vi "SMSD_CODE_CMD_REQUEST_cmd.vi"(8 "error in (no error)":errorcluster, 10 "Password":string="0123456789ABCDEF", 11 "SMSD in":refnum<class "SMSD Master.lvclass">) -> (0 "error out":errorcluster, 1 "PDU valid?":bool, 3 "SMSD out":refnum<class "SMSD Master.lvclass">)   [LabVIEW 2021, in "SMSD Master.lvclass"]
uses:
  SMSD Master.lvclass
  Data Unit/SMSD Data Unit/ERROR_OR_COMMANT_Type.ctl
  Data Unit/SMSD Data Unit/SMSD Data Unit.lvclass/SMSD Data Unit.ctl
  SMSD Master.lvclass/SMSD Master.ctl
  Transmission Data Unit/SMSD/SMSD ADU.lvclass/SMSD ADU.ctl
  Transmission Data Unit/SMSD/Write ADU Packet.vi
  Transmission Data Unit/SMSD/Read ADU Packet.vi
  Modbus_v121c/Network Interface/TCP Interface/TCP Shared Components/TCP Write.vi
  Data Unit/SMSD Data Unit/Flatten PDU.vi
  Data Unit/SMSD Data Unit/Unflatten to PDU.vi
  Modbus_v121c/Network Interface/TCP Interface/TCP Shared Components/TCP Read.vi
  <vilib>/Utility/error.llb/Clear Errors.vi
  Data Unit/SMSD Data Unit/SMSD Data Unit.lvclass
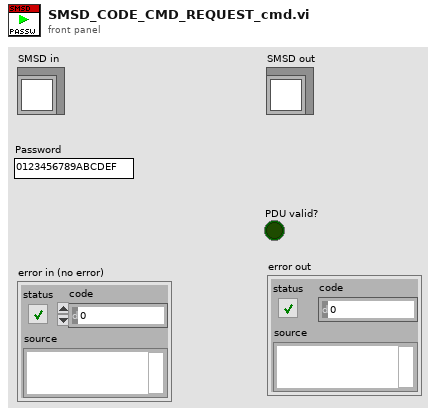
[diagram p1: front panel]
types:
  T1 = typedef "SMSD Data Unit.lvclass/ERROR_OR_COMMANT_Type.ctl" = enum8{"OK", "OK_ACCESS", "ERROR_ACCESS", "ERROR_ACCESS_TIMEOUT", "ERROR_XOR", "ERROR_NO_COMMAND", "ERROR_LEN", "ERROR_RANGE", "ERROR_WRITE", "ERROR_READ", "ERROR_PROGRAMS", "ERROR_WRITE_SETUP", "NO_NEXT", "END_PROGRAMS", "COMMAND_GET_STATUS_IN_EVENT", "COMMAND_GET_MODE", "COMMAND_GET_ABS_POS", "COMMAND_GET_EL_POS", "COMMAND_GET_SPEED", "COMMAND_GET_MIN_SPEED", "COMMAND_GET_MAX_SPEED", "COMMAND_GET_STACK", "STATUS_RELE_SET", "STATUS_RELE_CLR"}
  T2 = enum8{"CODE_CMD_REQUEST", "CODE_CMD_RESPONSE", "CODE_CMD_POWERSTEP01", "CODE_CMD_POWERSTEP01_W_MEM0", "CODE_CMD_POWERSTEP01_W_MEM1", "CODE_CMD_POWERSTEP01_W_MEM2", "CODE_CMD_POWERSTEP01_W_MEM3", "CODE_CMD_POWERSTEP01_R_MEM0", "CODE_CMD_POWERSTEP01_R_MEM1", "CODE_CMD_POWERSTEP01_R_MEM2", "CODE_CMD_POWERSTEP01_R_MEM3", "CODE_CMD_CONFIG_SET", "CODE_CMD_CONFIG_GET", "CODE_CMD_PASSWORD_SET", "CODE_CMD_ERROR_GET"}
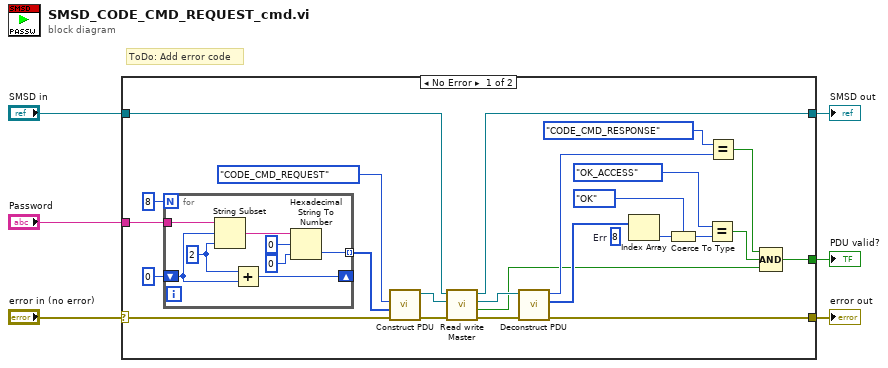
[diagram p0: block diagram]
diagram:
  # "ToDo: Add error code"
  n1 = case shown="No Error" "error in (no error)" {
    selector: "error in (no error)" -> [w30 w40]
    tunnel: [w20 w40] -> w6
    tunnel: "Password" -> [w17 _]
    tunnel: "SMSD in" -> [w29 w39]
    tunnel: [w24 w39] -> w3
    tunnel: [w7 _] -> w1
    frame No Error {
      (unwired) 8  # Err
      n2 = for {
        N: 8 -> [_]
        tunnel: w17 -> [w38]
        tunnel: [w34] -> w16 mode=indexing
        shift-right: [w33] -> _
        shift-left: 0 ("offset (0)") -> [w32]
        w31 = 2 ("y")
        n3 = String Subset(string=w38, offset (0)=w32, length (rest)=w31) -> (substring=w37:string)
        n4 = Add(x=w31, y=w32) -> (x+y=w33:i32)
        n5 = Hexadecimal String To Number(string=w37, offset=0, default (0uL)=u8 0 ("default (0 U32)")) -> (number=w34:u8)  [unwired: 1 out]
      }
      n6 = call "Construct PDU.vi"("error in"=w30, "DATA"=w16, "CMD_TYPE"=T2."CODE_CMD_REQUEST") -> ("error out"=w28:errorcluster, "SMSD data unit out"=w27:refnum<class "SMSD Data Unit.lvclass">)  [unwired: 7 in]
      n7 = call "Read write Master.vi"("error in (no error)"=w28, "ELAN data unit in"=w27, "ELAN master in"=w29) -> ("error out"=w25:errorcluster, "PDU valid?"=w8:bool, "ELAN data unit out"=w26:refnum<class "SMSD Data Unit.lvclass">, "ELAN master out"=w24:refnum<class "SMSD Master.lvclass">)  [unwired: 5 in]
      n8 = call "Deconstruct PDU.vi"("error in"=w25, "SMSD data unit in"=w26) -> ("error out"=w20:errorcluster, "DATA"=w12:u8[], "CMD_TYPE"=w23:T2)  [unwired: 7 in]
      n9 = Index Array(array=w12) -> (element=w11:u8)  [unwired: 1 in]
      n10 = Coerce To Type(0:w11, 1:ERROR_OR_COMMANT_Type."OK" ("Ring")) -> (2:w10:T1)
      n11 = Equal?(x=ERROR_OR_COMMANT_Type."OK_ACCESS" ("Ring"), y=w10) -> (x = y?=w9:bool)
      n12 = Equal?(x=T2."CODE_CMD_RESPONSE" ("CMD_TYPE"), y=w23) -> (x = y?=w21:bool)
      n13 = Compound Arithmetic op=AND(w21, w9, w8) -> (w7:bool)
    }
    frame Error {
    }
  }
  "error out" <- w6
  "SMSD out" <- w3
  "PDU valid?" <- w1
